vi "FlpLib ThreePhasePLL 2.vi"(0 "Vq":sgl, 1 "PLLgains":T3 {"proportional gain" step=0.125}, 3 "PLLrange":T2={"output high (Inf)"=inf, "output low (-Inf)"=-inf}, 5 "dT":sgl, 11 "Phase In":sgl, 12 "reset":bool) -> (4 "gridFrequency":sgl, 10 "PLLactions":T1, 15 "Phase Out":sgl)   [LabVIEW 2017]
uses:
  <vilib>/rvi/Analysis/control/PID/Typedef/niFpgaPID_PIGains.ctl
  <vilib>/rvi/Analysis/control/PID/Typedef/niFpgaPID_OutputRange.ctl
  <vilib>/rvi/Analysis/control/PID/Typedef/niFpgaPID_PIActions.ctl
  Control/PI_Controller/FlpLib PI_Controller 2.vi
  <userlib>/_NI FLP Library/FPGA/outsideSCTL/FlpLib Multiply Shared Instance 2.vi
  <userlib>/_NI FLP Library/FPGA/outsideSCTL/FlpLib Add Shared Instance 2.vi
  <userlib>/_NI FLP Library/FPGA/outsideSCTL/FlpLib Subtract Shared Instance 2.vi
  <userlib>/_NI FLP Library/FPGA/outsideSCTL/FlpLib Greater Than Shared Instance 2.vi
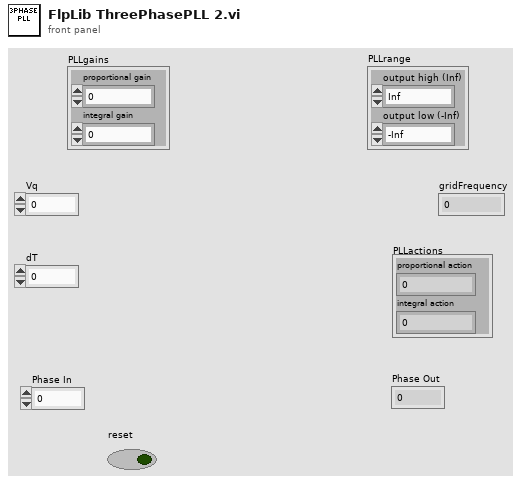
[diagram p1: front panel]
types:
  T1 = typedef "niFpgaPID_PIActions.ctl" = cluster{"proportional action":sgl, "integral action":sgl}
  T2 = typedef "niFpgaPID_OutputRange.ctl" = cluster{"output high (Inf)":sgl, "output low (-Inf)":sgl}
  T3 = typedef "niFpgaPID_PIGains.ctl" = cluster{"proportional gain":sgl, "integral gain":sgl}
  T4 = typedef "niFpgaPID_PIState.ctl" = cluster{"uI(k-1)":sgl, "e(k-1)":sgl, "output (k-1)":sgl}
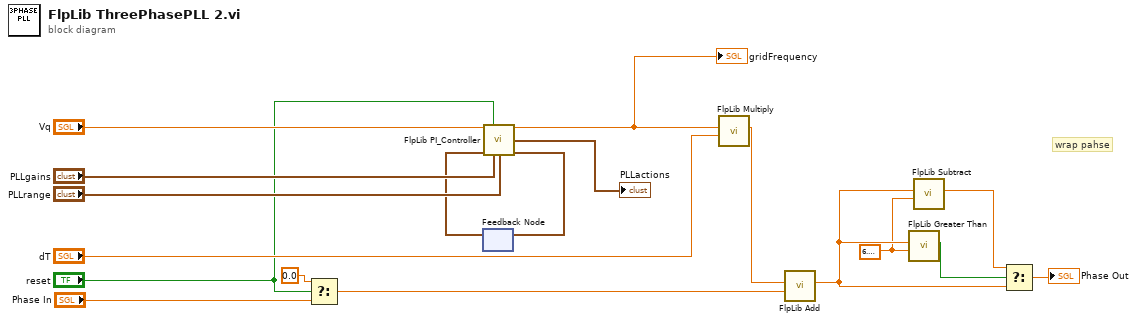
[diagram p0: block diagram]
diagram:
  w4 = sgl 6.2831855
  # "wrap pahse"
  n1 = Select(t=sgl 0.0, s="reset", f="Phase In") -> (s? t:f=w10:sgl)
  n2 = feedback #1() -> (w1:T4)  [unwired: 1 in]
  n3 = call-poly "FlpLib PI_Controller.vi"("error"="Vq", "reset? (F)"="reset", "state in"=w1, "gains"="PLLgains", "output range"="PLLrange") -> ("output"=w3:sgl, "actions"=→"PLLactions":T1, "state out"=w18:T4)  [unwired: 7 in, 1 out]
  "gridFrequency" <- w3
  n4 = feedback-in #1(w18) -> ()
  n5 = call-poly <userlib>:"FlpLib Multiply.vi"("y"="dT", "x"=w3) -> ("x*y"=w11:sgl)  [unwired: 5 in]
  n6 = call-poly <userlib>:"FlpLib Add.vi"("y"=w10, "x"=w11) -> ("x+y"=w9:sgl)  [unwired: 5 in]
  n7 = call-poly <userlib>:"FlpLib Greater Than.vi"("y"=w4, "x"=w9) -> ("x > y?"=w14:bool)  [unwired: 5 in]
  n8 = call-poly <userlib>:"FlpLib Subtract.vi"("y"=w4, "x"=w9) -> ("x-y"=w8:sgl)  [unwired: 5 in]
  n9 = Select(t=w8, s=w14, f=w9) -> (s? t:f=→"Phase Out":sgl)
